vi "SMSD_powerstep01_cmd.vi"(8 "error in (no error)":errorcluster, 9 "DATA (0)":u32 format="%x", 10 "COMMAND (END)":T1(ring), 11 "SMSD in":refnum<class "SMSD Master.lvclass">) -> (0 "error out":errorcluster, 1 "PDU valid?":bool, 2 "data":u8[](array[numeric]), 3 "SMSD out":refnum<class "SMSD Master.lvclass">)   [LabVIEW 2021, in "SMSD Master.lvclass"]
uses:
  SMSD Master.lvclass
  Data Unit/SMSD Data Unit/SMSD Data Unit.lvclass/SMSD Data Unit.ctl
  SMSD Master.lvclass/SMSD Master.ctl
  Transmission Data Unit/SMSD/SMSD ADU.lvclass/SMSD ADU.ctl
  Transmission Data Unit/SMSD/Write ADU Packet.vi
  Transmission Data Unit/SMSD/Read ADU Packet.vi
  Modbus_v121c/Network Interface/TCP Interface/TSC/TCP Write.vi
  Data Unit/SMSD Data Unit/Flatten PDU.vi
  Data Unit/SMSD Data Unit/Unflatten to PDU.vi
  Modbus_v121c/Network Interface/TCP Interface/TSC/TCP Read.vi
  <vilib>/Utility/error.llb/Clear Errors.vi
  Data Unit/SMSD Data Unit/SMSD Data Unit.lvclass
  Devices/SMSD/SMSD.lvclass
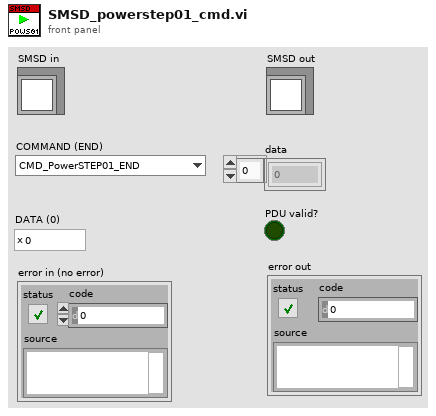
[diagram p1: front panel]
types:
  T1 = enum8{"CMD_PowerSTEP01_END", "CMD_PowerSTEP01_GET_SPEED", "CMD_PowerSTEP01_STATUS_IN_EVENT", "CMD_PowerSTEP01_SET_MODE", "CMD_PowerSTEP01_GET_MODE", "CMD_PowerSTEP01_SET_MIN_SPEED", "CMD_PowerSTEP01_SET_MAX_SPEED", "CMD_PowerSTEP01_SET_ACC", "CMD_PowerSTEP01_SET_DEC", "CMD_PowerSTEP01_SET_FS_SPEED", "CMD_PowerSTEP01_SET_MASK_EVENT", "CMD_PowerSTEP01_GET_ABS_POS", "CMD_PowerSTEP01_GET_EL_POS", "CMD_PowerSTEP01_GET_STATUS_AND_CLR", "CMD_PowerSTEP01_RUN_F", "CMD_PowerSTEP01_RUN_R", "CMD_PowerSTEP01_MOVE_F", "CMD_PowerSTEP01_MOVE_R", "CMD_PowerSTEP01_GO_TO_F", "CMD_PowerSTEP01_GO_TO_R", "CMD_PowerSTEP01_GO_UNTIL_F", "CMD_PowerSTEP01_GO_UNTIL_R", "CMD_PowerSTEP01_SCAN_ZERO_F", "CMD_PowerSTEP01_SCAN_ZERO_R", "CMD_PowerSTEP01_SCAN_LABEL_F", "CMD_PowerSTEP01_SCAN_LABEL_R", "CMD_PowerSTEP01_GO_ZERO", "CMD_PowerSTEP01_GO_LABEL", "CMD_PowerSTEP01_GO_TO", "CMD_PowerSTEP01_RESET_POS", "CMD_PowerSTEP01_RESET_POWERSTEP01", "CMD_PowerSTEP01_SOFT_STOP", "CMD_PowerSTEP01_HARD_STOP", "CMD_PowerSTEP01_SOFT_HI_Z", "CMD_PowerSTEP01_HARD_HI_Z", "CMD_PowerSTEP01_SET_WAIT", "CMD_PowerSTEP01_SET_RELE", "CMD_PowerSTEP01_CLR_RELE", "CMD_PowerSTEP01_GET_RELE", "CMD_PowerSTEP01_WAIT_IN0", "CMD_PowerSTEP01_WAIT_IN1", "CMD_PowerSTEP01_GOTO_PROGRAM", "CMD_PowerSTEP01_GOTO_PROGRAM_IF_IN0", "CMD_PowerSTEP01_GOTO_PROGRAM_IF_IN1", "CMD_PowerSTEP01_LOOP_PROGRAM", "CMD_PowerSTEP01_CALL_PROGRAM", "CMD_PowerSTEP01_RETURN_PROGRAM", "CMD_PowerSTEP01_START_PROGRAM_MEM0", "CMD_PowerSTEP01_START_PROGRAM_MEM1", "CMD_PowerSTEP01_START_PROGRAM_MEM2", "CMD_PowerSTEP01_START_PROGRAM_MEM3", "CMD_PowerSTEP01_STOP_PROGRAM_MEM", "CMD_PowerSTEP01_STEP_CLOCK", "CMD_PowerSTEP01_STOP_USB", "CMD_PowerSTEP01_GET_MIN_SPEED", "CMD_PowerSTEP01_GET_MAX_SPEED", "CMD_PowerSTEP01_GET_STACK", "CMD_PowerSTEP01_GOTO_PROGRAM_IF_ZERO", "CMD_PowerSTEP01_GOTO_PROGRAM_IF_IN_ZERO", "CMD_PowerSTEP01_WAIT_CONTINUE", "CMD_PowerSTEP01_SET_WAIT_2", "CMD_PowerSTEP01_SCAN_MARK2_F", "CMD_PowerSTEP01_SCAN_MARK2_R"}
  T2 = enum8{"CODE_CMD_REQUEST", "CODE_CMD_RESPONSE", "CODE_CMD_POWERSTEP01", "CODE_CMD_POWERSTEP01_W_MEM0", "CODE_CMD_POWERSTEP01_W_MEM1", "CODE_CMD_POWERSTEP01_W_MEM2", "CODE_CMD_POWERSTEP01_W_MEM3", "CODE_CMD_POWERSTEP01_R_MEM0", "CODE_CMD_POWERSTEP01_R_MEM1", "CODE_CMD_POWERSTEP01_R_MEM2", "CODE_CMD_POWERSTEP01_R_MEM3", "CODE_CMD_CONFIG_SET", "CODE_CMD_CONFIG_GET", "CODE_CMD_PASSWORD_SET", "CODE_CMD_ERROR_GET"}
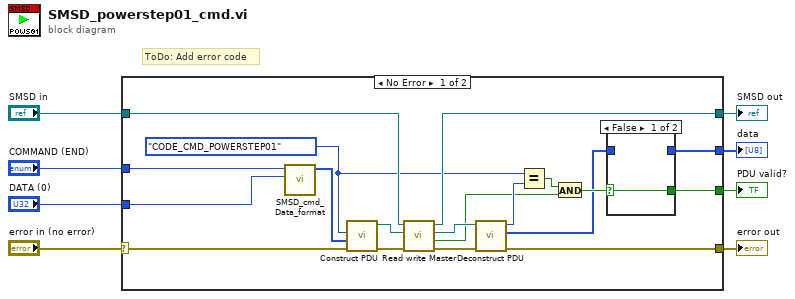
[diagram p0: block diagram]
diagram:
  # "ToDo: Add error code"
  n1 = case shown="No Error" "error in (no error)" {
    selector: "error in (no error)" -> [w24 w32]
    tunnel: [w11 _] -> w8
    tunnel: [w9 w32] -> w7
    tunnel: "COMMAND (END)" -> [w27 _]
    tunnel: "SMSD in" -> [w23 w31]
    tunnel: [w18 w31] -> w4
    tunnel: "DATA (0)" -> [w26 _]
    tunnel: [w10 _] -> w1
    frame No Error {
      w16 = T2."CODE_CMD_POWERSTEP01" ("CMD_TYPE")
      n2 = call "SMSD_cmd_Data_format.vi"("DATA (0)"=w26, "COMMAND (END)"=w27) -> ("SMSD_CMD_out"=w25:u8[])  [unwired: 9 in]
      n3 = call "Construct PDU.vi"("error in"=w24, "DATA"=w25, "CMD_TYPE"=w16) -> ("error out"=w22:errorcluster, "SMSD data unit out"=w21:refnum<class "SMSD Data Unit.lvclass">)  [unwired: 7 in]
      n4 = call "Read write Master.vi"("error in (no error)"=w22, "ELAN data unit in"=w21, "ELAN master in"=w23) -> ("error out"=w19:errorcluster, "PDU valid?"=w14:bool, "ELAN data unit out"=w20:refnum<class "SMSD Data Unit.lvclass">, "ELAN master out"=w18:refnum<class "SMSD Master.lvclass">)  [unwired: 5 in]
      n5 = call "Deconstruct PDU.vi"("error in"=w19, "SMSD data unit in"=w20) -> ("error out"=w9:errorcluster, "DATA"=w12:u8[], "CMD_TYPE"=w17:T2)  [unwired: 7 in]
      n6 = Equal?(x=w16, y=w17) -> (x = y?=w15:bool)
      n7 = And(x=w15, y=w14) -> (x .and. y?=w13:bool)
      n8 = case shown="False" w13 {
        selector: w13 -> [w28 w29]
        tunnel: w12 -> [_ w30]
        tunnel: [_ w30] -> w11
        tunnel: [w28 w29] -> w10
        frame False {
        }
        frame True {
        }
      }
    }
    frame Error {
    }
  }
  "data" <- w8
  "error out" <- w7
  "SMSD out" <- w4
  "PDU valid?" <- w1
